vi "direction.vi"(1 "反向":bool=TRUE) -> (0 "指令":string)   [LabVIEW 2018]
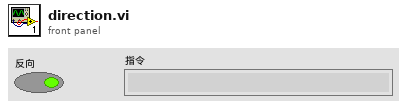
[diagram p1: front panel]
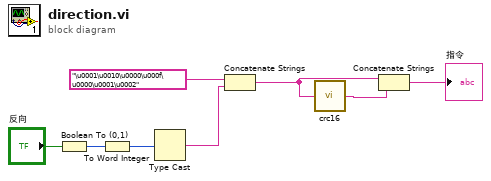
[diagram p0: block diagram]
diagram:
  n1 = Boolean To (0,1)(Boolean="反向") -> (0, 1=w1:i16)
  n2 = To Word Integer(number=w1) -> (16bit integer=w3:i16)
  n3 = Type Cast(x=w3) -> (*(type *) &x=w4:string)  [unwired: 1 in]
  n4 = Concatenate Strings("\u0001\u0010\u0000\u000f\u0000\u0001\u0002" ("字符串"), w4) -> (w6:string)
  n5 = call "crc16.vi"("message"=w6) -> ("CRC16"=w7:string)  [unwired: 4 in]
  n6 = Concatenate Strings(w6, w7) -> (→"指令":string)
